vi "Stop Core.vi"(10 "final error code":i32, 11 "BNT_DAQmx_MCSV-Ctr2Freq in":refnum<class "BNT_DAQmx-MCSV-Ctr2Freq.lvclass">) -> (3 "BNT_DAQmx_MCSV-Ctr2Freq out":refnum<class "BNT_DAQmx-MCSV-Ctr2Freq.lvclass">)   [LabVIEW 2017, in "BNT_DAQmx.lvlib" / "BNT_DAQmx-MCSV-Ctr2Freq.lvclass"]
doc: "(<B>Filename</B>: Actor Framework.lvlib:Actor.lvclass:Stop Core.vi)\n\nDefines what the actor does before it stops. Use the <B>final error code</B> input to determine whether the actor shut down in response to an error.\n\nBy default, this method does nothing. A descendant class may override it to define behavior, such as shutting down any processes the actor initiated in its override of the Actor Core method."
uses:
  BNT_DAQmx-MCSV-Ctr2Freq.lvclass
  BNT_DAQmx-MCSV-Ctr2Freq.lvclass/BNT_DAQmx-MCSV-Ctr2Freq.ctl
  BNT_DAQmx-MCSV/BNT_DAQmx-MCSV.lvclass
  CSPP_Core/Classes/CS++ProcessVariables/PVConnection/PVConnection.lvclass
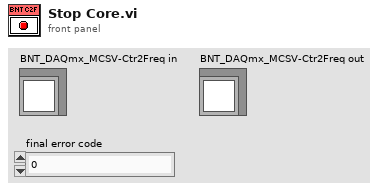
[diagram p1: front panel]
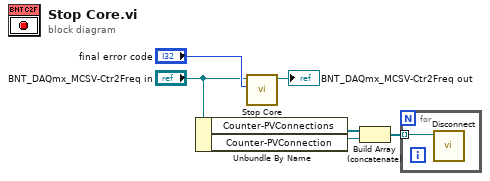
[diagram p0: block diagram]
diagram:
  n1 = Unbundle By Name("BNT_DAQmx_MCSV-Ctr2Freq in") -> ("Counter-PVConnections"=w2:refnum<class "PVConnection.lvclass">[], "Counter-PVConnection"=w1:refnum<class "PVConnection.lvclass">)
  n2 = call-parent "Stop Core.vi"("final error code"="final error code", "BNT_DAQmx-MCSV in"="BNT_DAQmx_MCSV-Ctr2Freq in") -> ("BNT_DAQmx-MCSV out"=→"BNT_DAQmx_MCSV-Ctr2Freq out":refnum<class "BNT_DAQmx-MCSV-Ctr2Freq.lvclass">)  [unwired: 9 in]
  n3 = Build Array (concatenate)(w2, w1) -> (w4:refnum<class "PVConnection.lvclass">[])
  n4 = for {
    tunnel: w4 -> [w7] mode=indexing
    n5 = call "Disconnect.vi"("PVConnection in"=w7) -> ()  [unwired: 9 in, 2 out]
  }
